vi "even&odd_subvi.vi"(2 "String 2":string, 3 "Numeric":dbl, 4 "String":string) -> (0 "s? t:f":string, 1 "even":bool)   [LabVIEW 2020]
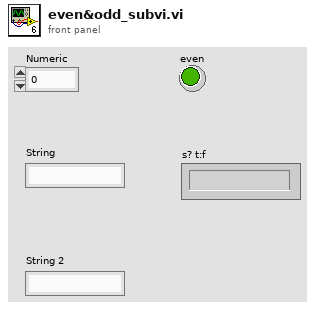
[diagram p1: front panel]
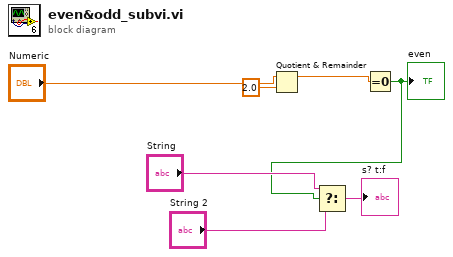
[diagram p0: block diagram]
diagram:
  n1 = Quotient & Remainder(x="Numeric", y=2.0) -> (x-y*floor(x/y)=w3:dbl)  [unwired: 1 out]
  n2 = Equal To 0?(x=w3) -> (x = 0?=w4:bool)
  "even" <- w4
  n3 = Select(t="String", s=w4, f="String 2") -> (s? t:f=→"s? t:f":string)
